vi "Publish State.vi"(9 "result allocation in":T1, 11 "Sequencer Module runtime in":refnum<class "Sequencer Module runtime.lvclass">) -> (1 "result allocation out":T1, 3 "Sequencer Module runtime out":refnum<class "Sequencer Module runtime.lvclass">)   [LabVIEW 2015, in "Sequencer Module runtime.lvclass"]
uses:
  Sequencer Module runtime.lvclass
  <vilib>/NI/Tag Bus/table/data table.ctl
  Sequencer Module runtime.lvclass/Sequencer Module runtime.ctl
  <vilib>/NI/Tag Bus/table/data polymorphs/write one/write I32.vi
  <vilib>/NI/Tag Bus/table/data polymorphs/write one/write String.vi
  <vilib>/NI/Tag Bus/table/data table.lvlib
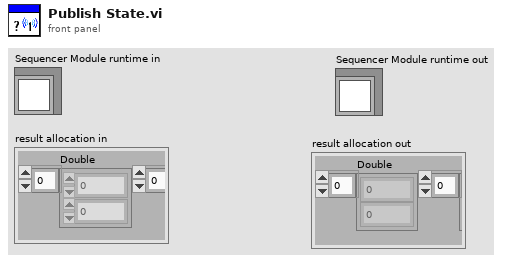
[diagram p1: front panel]
types:
  T1 = typedef "tag bus.lvlib/data table.lvlib/data table.ctl" = cluster{"Double":dbl[], "Single":sgl[], "I64":i64[], "I32":i32[], "I16":i16[], "I8":i8[], "U64":u64[], "U32":u32[], "U16":u16[], "U8":u8[], "Boolean":bool[], "String":string[], "Array of Double":cluster{"DBL Array":dbl[]}[], "Array of Single":cluster{"SGL Array":sgl[]}[], "Array of I64":cluster{"I64 Array":i64[]}[], "Array of I32":cluster{"I32 Array":i32[]}[], "Array of I16":cluster{"I16 Array":i16[]}[], "Array of I8":cluster{"I8 Array":i8[]}[], "Array of U64":cluster{"U64 Array":u64[]}[], "Array of U32":cluster{"U32 Array":u32[]}[], "Array of U16":cluster{"U16 Array":u16[]}[], "Array of U8":cluster{"U8 Array":u8[]}[], "Array of Boolean":cluster{"Boolean Array":bool[]}[], "Array of String":cluster{"String Array":string[]}[]}
  T2 = typedef "Sequencer Module runtime.lvclass/Sequencer State Index.ctl" = cluster{"Sequencer State":i32, "Active Sequence Name":i32, "Active Sequence Index":i32, "Active Step":i32, "Active Step State":i32}
  T3 = typedef "Sequencer Module runtime.lvclass/Sequencer State Cluster.ctl" = cluster{"Sequencer State":T4, "Sequence #":i32, "Active Sequence Name":string, "Active Step":i32, "Step State":T5}
  T4 = typedef "Sequencer Module runtime.lvclass/Sequencer State Enum.ctl" = enum16{"Iddle", "Running", "Paused"}
  T5 = typedef "Step.lvclass/StepState.ctl" = cluster{"Step State":T6, "Flow Control":T7, "Jump Index":i32}
  T6 = typedef "Step.lvclass/Step State Enum.ctl" = enum16{"Start", "Skipped", "Completed", "Running", "Aborted"}
  T7 = typedef "Step.lvclass/Step Flow Control.ctl" = enum16{"Next Step", "Jump"}
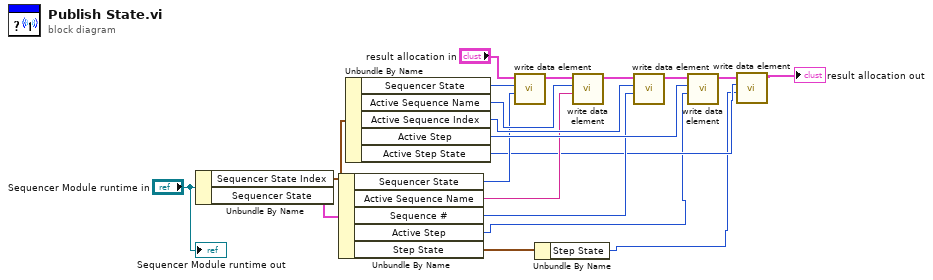
[diagram p0: block diagram]
diagram:
  n1 = Unbundle By Name("Sequencer Module runtime in") -> ("Sequencer State Index"=w19:T2, "Sequencer State"=w10:T3)
  n2 = Unbundle By Name(w10) -> ("Sequencer State"=w9:T4, "Active Sequence Name"=w8:string, "Sequence #"=w7:i32, "Active Step"=w1:i32, "Step State"=w3:T5)
  n3 = Unbundle By Name(w19) -> ("Sequencer State"=w18:i32, "Active Sequence Name"=w17:i32, "Active Sequence Index"=w16:i32, "Active Step"=w11:i32, "Active Step State"=w4:i32)
  n4 = call-poly <vilib>:"write data element.vi"("value"=w9, "index"=w18, "data table in"="result allocation in") -> ("data table out"=w14:T1)  [unwired: 8 in]
  n5 = Unbundle By Name(w3) -> ("Step State"=w2:T6)
  n6 = call-poly <vilib>:"write data element.vi"("value"=w8, "index"=w17, "data table in"=w14) -> ("data table out"=w13:T1)  [unwired: 8 in]
  n7 = call-poly <vilib>:"write data element.vi"("value"=w7, "index"=w16, "data table in"=w13) -> ("data table out"=w12:T1)  [unwired: 8 in]
  n8 = call-poly <vilib>:"write data element.vi"("value"=w1, "index"=w11, "data table in"=w12) -> ("data table out"=w6:T1)  [unwired: 8 in]
  n9 = call-poly <vilib>:"write data element.vi"("value"=w2, "index"=w4, "data table in"=w6) -> ("data table out"=→"result allocation out":T1)  [unwired: 8 in]
  "Sequencer Module runtime out" <- "Sequencer Module runtime in"
